vi "Waveform Data Logger Main Page.vi"(8 "error in (no error)":errorcluster, 11 "Node Ptr":T1 format="%.0x") -> (0 "error out":errorcluster)   [LabVIEW 2015, in "Waveform Data Logger System Explorer.lvlib"]
uses:
  Waveform Data Logger System Explorer.lvlib
  <vilib>/NI Veristand/Custom Device API/Custom Device Item Ref.ctl
  Shared/Globals/Global GUIDs.vi
  Shared/Globals/Property Strings.vi
  <vilib>/NI Veristand/Custom Device API/Get Item Property (Boolean).vi
  <vilib>/NI Veristand/Custom Device API/Get Item Property (I32).vi
  <vilib>/NI Veristand/Custom Device Tools/Custom Device Utility Library/NI VeriStand - Search for All Items by GUID.vi
  Shared/Globals/Default Values.vi
  <vilib>/NI Veristand/Custom Device API/Set Item Property (Boolean).vi
  <vilib>/NI Veristand/Custom Device API/Set Item Property (I32).vi
  <vilib>/NI VeriStand/Custom Device API/Custom Device API.lvlib
  <vilib>/NI VeriStand/Custom Device Tools/Custom Device Utility Library/Custom Device Utility Library.lvlib
  Shared/Waveform Data Logger Shared.lvlib
panel:
  in  "Q Size":i32=5 format="%d elements per waveform"
  in  "Auto Q Size":bool
  out "Version":string
  in  "Header 2":cluster{"Section Name":string}={"Section Name"="Waveform Log Files"}
  in  "Remove":bool
  in  "TDMS Log Files":i32(listbox)
  in  "Add File":bool
  in  "Header":cluster{"Section Name":string}={"Section Name"="Waveform Data Logger Specification"}
  out "Name":string
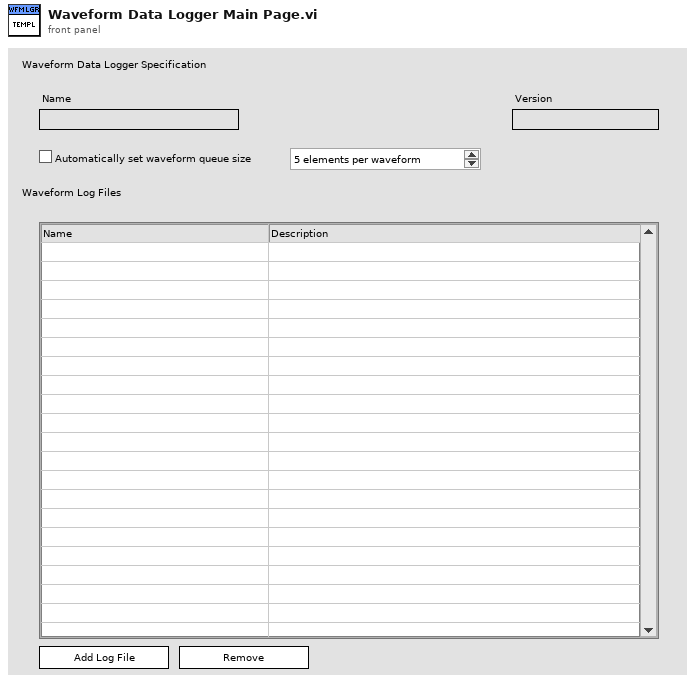
[diagram p1: front panel]
types:
  T1 = typedef "Custom Device API.lvlib/Custom Device Item Ref.ctl" = u64
  T2 = enum8{"Enabled", "Disabled", "Disabled and Grayed Out"}
  T3 = typedef "Custom Device API.lvlib/Custom Device Item Info.ctl" = cluster{"Name":string, "Is Channel":bool, "GUID":string, "Is Waveform":bool}
  T4 = typedef "Custom Device API.lvlib/Custom Device Commands.ctl" = enum16{"Default", "Item renamed", "Shutdown", "Dynamic button pressed"}
  T5 = typedef "LVRowAndColumnTypeDef.ctl" = cluster{"Row":i32, "Column":i32}
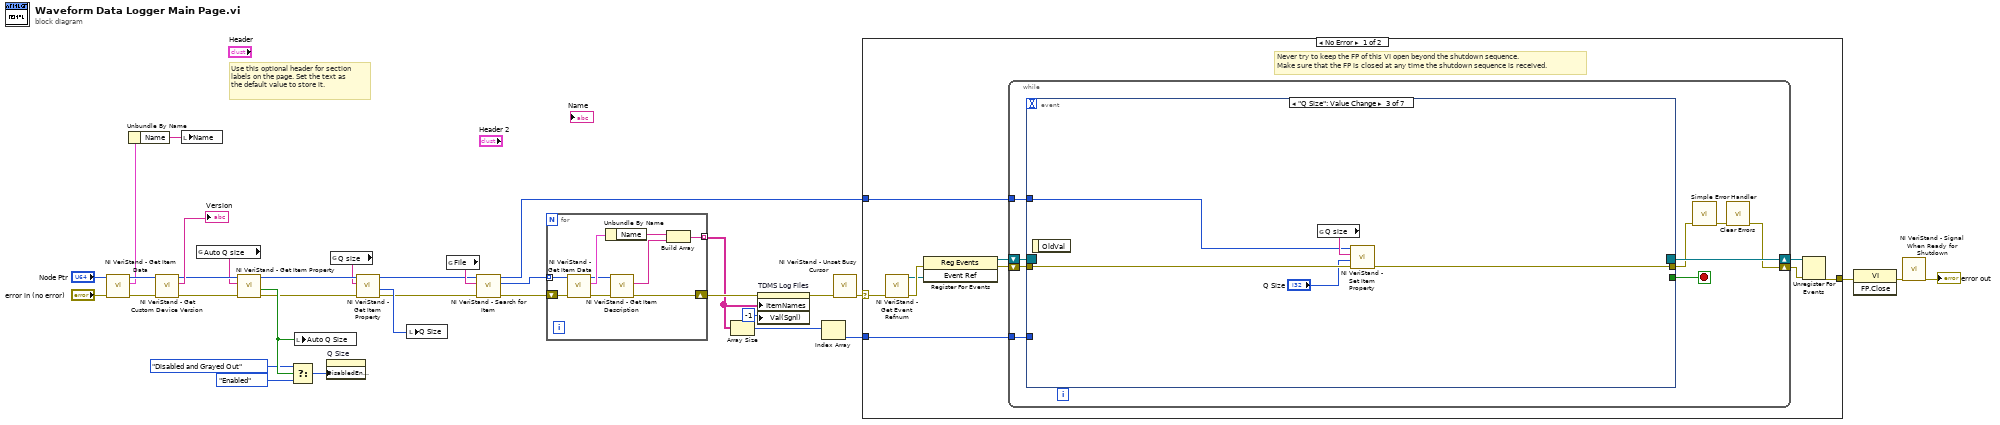
[diagram p0: block diagram]
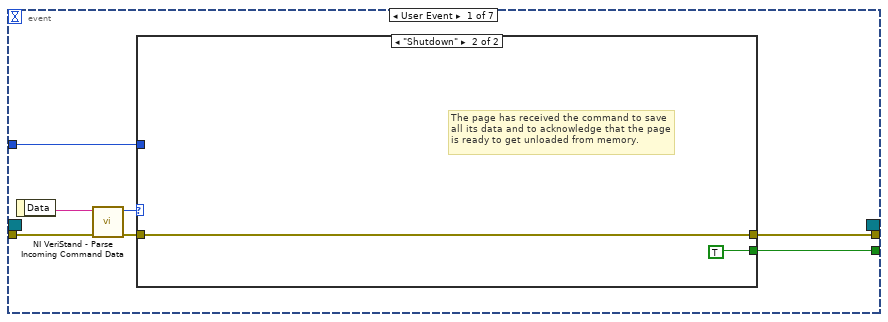
[diagram p2: hidden frame]
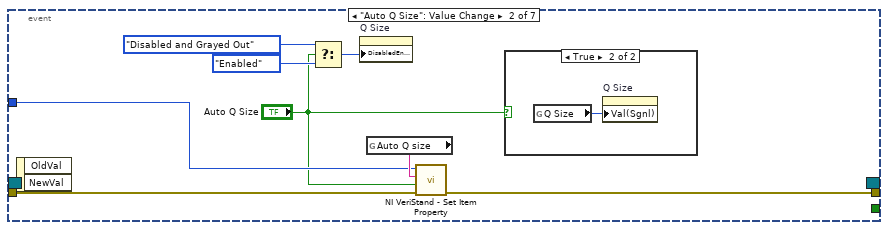
[diagram p4: hidden frame]
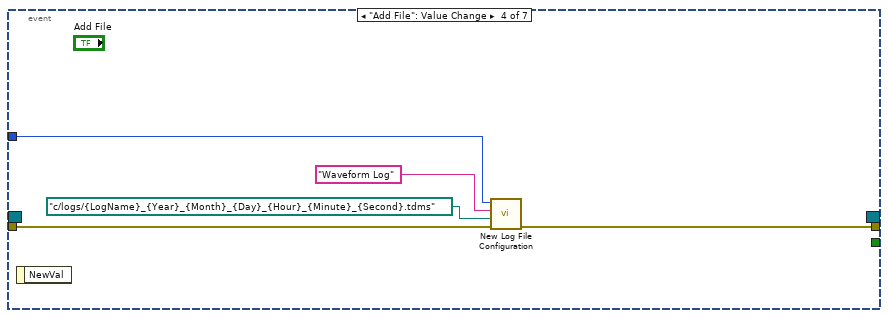
[diagram p6: hidden frame]
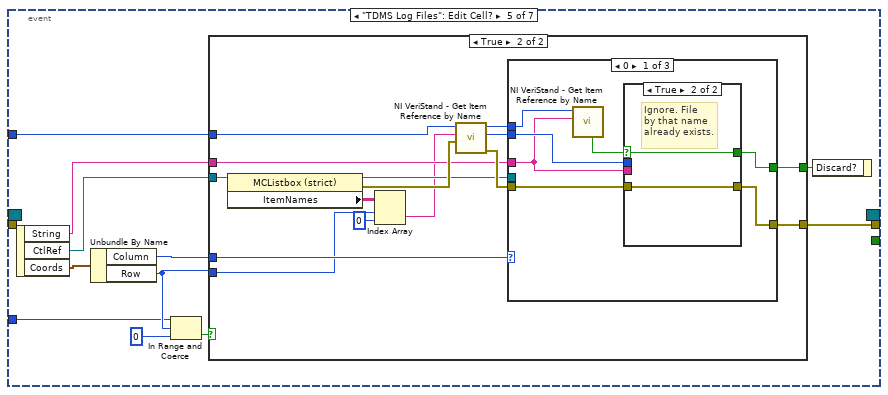
[diagram p7: hidden frame]
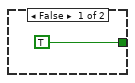
[diagram p8: hidden frame]
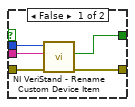
[diagram p9: hidden frame]
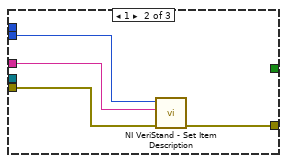
[diagram p10: hidden frame]
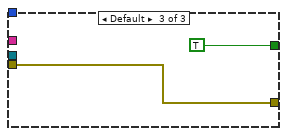
[diagram p11: hidden frame]
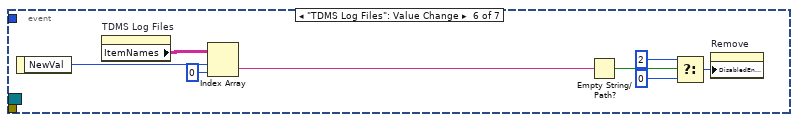
[diagram p12: hidden frame]
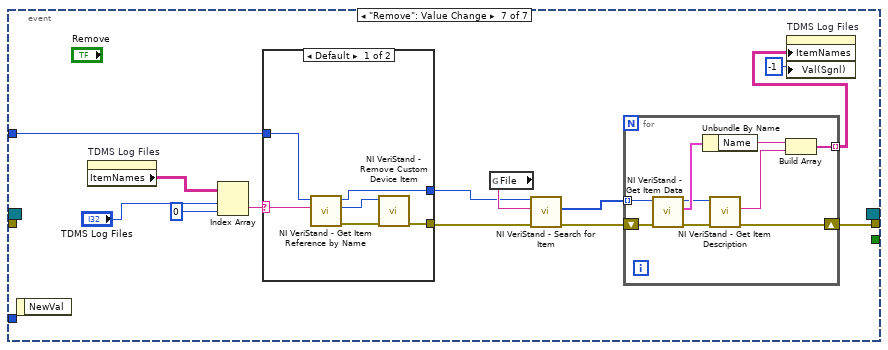
[diagram p13: hidden frame]
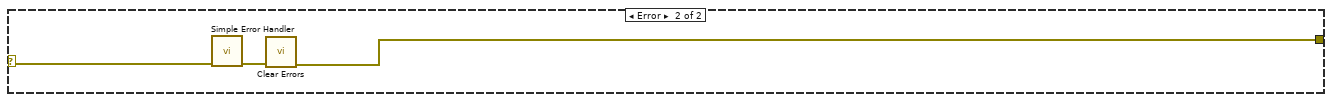
[diagram p15: hidden frame]
diagram:
  # "Use this optional header for section labels on the page. Set the text as the default value to store it."
  n1 = call <vilib>:"NI VeriStand - Get Item Data.vi"("error in (no error)"="error in (no error)", "Item Ref in"="Node Ptr") -> ("error out"=w16:errorcluster, "Item Info"=w1:T3, "Item Ref out"=w17:T1)  [unwired: 7 out]
  n2 = Unbundle By Name(w1) -> ("Name"=w31:string)
  n3 = call <vilib>:"NI VeriStand - Get Custom Device Version.vi"("error in (no error)"=w16, "Device Ref in"=w17) -> ("error out"=w13:errorcluster, "Value"=→"Version":string, "Device Ref out"=w14:T1)  [unwired: 7 in]
  n4 = local write "Name"(w31) -> ()
  n5 = global read "Property Strings.vi" "Auto Q size"() -> (w12:string)
  n6 = call-poly <vilib>:"NI VeriStand - Get Item Property.vi"("error in (no error)"=w13, "Property Name"=w12, "Item Ref in"=w14) -> ("error out"=w6:errorcluster, "Value"=w11:bool, "Item Ref out"=w7:T1)  [unwired: 5 in, 1 out]
  n7 = Select(t=T2."Disabled and Grayed Out" ("Disabled"), s=w11, f=T2."Enabled" ("Disabled")) -> (s? t:f=w8:T2)
  n8 = local write "Auto Q Size"(w11) -> ()
  n9 = property on="Q Size" class="DigNum (strict)"("DisabledEnum"=w8) -> ()  [unwired: 2 in, 2 out]
  n10 = global read "Property Strings.vi" "Q size"() -> (w5:string)
  n11 = call-poly <vilib>:"NI VeriStand - Get Item Property.vi"("error in (no error)"=w6, "Property Name"=w5, "Item Ref in"=w7) -> ("error out"=w3:errorcluster, "Value"=w4:i32, "Item Ref out"=w2:T1)  [unwired: 5 in, 1 out]
  n12 = local write "Q Size"(w4) -> ()
  n13 = global read "Global GUIDs.vi" "File"() -> (w20:string)
  n14 = call-poly <vilib>:"NI VeriStand - Search for Item.vi"("error in"=w3, "Item GUID"=w20, "Section Ref in"=w2) -> ("error out"=w24:errorcluster, "Item Refs"=w23:T1[], "Section Ref out"=w22:T1)  [unwired: 5 in, 1 out]
  n15 = for {
    tunnel: w23 -> [w42] mode=indexing
    tunnel: [w38] -> w27 mode=indexing
    shift-right: [w37] -> w30
    shift-left: w24 -> [w43]
    n16 = call <vilib>:"NI VeriStand - Get Item Data.vi"("error in (no error)"=w43, "Item Ref in"=w42) -> ("error out"=w35:errorcluster, "Item Info"=w41:T3, "Item Ref out"=w36:T1)  [unwired: 6 in, 1 out]
    n17 = Unbundle By Name(w41) -> ("Name"=w40:string)
    n18 = call <vilib>:"NI VeriStand - Get Item Description.vi"("error in (no error)"=w35, "Item Ref in"=w36) -> ("error out"=w37:errorcluster, "Description"=w39:string)  [unwired: 6 in, 2 out]
    n19 = Build Array(w40, w39) -> (w38:string[])
  }
  n20 = Array Size(array=w27) -> (size(s)=w26:i32[])
  n21 = property on="TDMS Log Files" class="MCListbox (strict)"(error in=w30, "ItemNames"=w27, "Val(Sgnl)"=-1 ("Value (Signaling)")) -> (error out=w28:errorcluster)  [unwired: 1 in, 1 out]
  n22 = Index Array(array=w26) -> (element=w25:i32)  [unwired: 1 in]
  n23 = call <vilib>:"NI VeriStand - Unset Busy Cursor.vi"("error in (no error)"=w28) -> ("error out"=w32:errorcluster)  [unwired: 10 out]
  n24 = case shown="No Error" w32 {
    selector: w32 -> [w45 w178]
    tunnel: [w50 w176] -> w19
    tunnel: w22 -> [w46 _]
    tunnel: w25 -> [w44 _]
    frame No Error {
      # "Never try to keep the FP of this VI open beyond the shutdown sequence.\nMake sure that the FP is closed at any time the shutdown sequence is received."
      n25 = call <vilib>:"NI VeriStand - Get Event Refnum.vi"("error in (no error)"=w45) -> ("error out"=w53:errorcluster, "Event Ref"=w49:refnum<user-event>)  [unwired: 9 out]
      n26 = register-events(error in=w53, w49) -> (reference out=w47:refnum<event-registration>, error out=w48:errorcluster)  [unwired: 1 in]
      n27 = while {
        tunnel: w46 -> [w59]
        shift-right: [w56] -> w51
        shift-left: w48 -> [w61]
        shift-right: [w62] -> w52
        shift-left: w47 -> [w54]
        tunnel: w44 -> [w55]
        stop <- w60 stop-if-true
        n28 = event shown="[2] \"Q Size\": Value Change" {
          selector: w54 -> [_ _ _ _ _ _ _]
          dyn-events: [_ _ _ _ _ _ _] -> w62
          timeout: _ -> [_ _ _ _ _ _ _]
          tunnel: w61 -> [w69 w79 w84 w90 _ _ _]
          tunnel: [w65 _ _ _ _ _ _] -> w60
          tunnel: [w64 w77 w82 w89 w98 _ w149] -> w58
          tunnel: w59 -> [w63 w78 w85 w91 w93 _ w157]
          tunnel: w55 -> [_ _ _ _ w92 _ _]
          event User Event {
            n29 = event-data() -> ("Data"=w68:string)  [unwired: 1 out]
            n30 = call <vilib>:"NI VeriStand - Parse Incoming Command Data.vi"("error in (no error)"=w69, "Incoming data"=w68) -> ("error out"=w67:errorcluster, "Action"=w66:T4)  [unwired: 8 out]
            n31 = case shown="\"Shutdown\"" w66 {
              tunnel: w67 -> [w70 w71]
              tunnel: [_ TRUE] -> w65
              tunnel: [w70 w71] -> w64
              tunnel: w63 -> [_ _]
              frame "Default", Default {
              }
              frame "Shutdown" {
                # "The page has received the command to save all its data and to acknowledge that the page is ready to get unloaded from memory."
              }
            }
          }
          event "Auto Q Size": Value Change {
            n32 = event-data() -> ()  [unwired: 3 out]
            n33 = Select(t=T2."Disabled and Grayed Out" ("Disabled"), s="Auto Q Size", f=T2."Enabled" ("Disabled")) -> (s? t:f=w76:T2)
            n34 = property on="Q Size" class="DigNum (strict)"("DisabledEnum"=w76) -> ()  [unwired: 2 in, 2 out]
            n35 = global read "Property Strings.vi" "Auto Q size"() -> (w80:string)
            n36 = call-poly <vilib>:"NI VeriStand - Set Item Property.vi"("error in (no error)"=w79, "Value"="Auto Q Size", "Property Name"=w80, "Item Ref in"=w78) -> ("error out"=w77:errorcluster)  [unwired: 5 in, 2 out]
            n37 = case shown="True" "Auto Q Size" {
              frame False {
              }
              frame True {
                n38 = global read "Default Values.vi" "Q Size"() -> (w81:i32)
                n39 = property on="Q Size" class="DigNum (strict)"("Val(Sgnl)"=w81) -> ()  [unwired: 2 in, 2 out]
              }
            }
          }
          event "Q Size": Value Change {
            n40 = event-data() -> ()  [unwired: 2 out]
            n41 = global read "Property Strings.vi" "Q size"() -> (w86:string)
            n42 = call-poly <vilib>:"NI VeriStand - Set Item Property.vi"("error in (no error)"=w84, "Value"="Q Size", "Property Name"=w86, "Item Ref in"=w85) -> ("error out"=w82:errorcluster)  [unwired: 5 in, 2 out]
          }
          event "Add File": Value Change {
            n43 = event-data() -> ()  [unwired: 2 out]
            n44 = call "New Log File Configuration.vi"("error in (no error)"=w90, "Default Path"=path "c:/logs/{LogName}_{Year}_{Month}_{Day}_{Hour}_{Minute}_{Second}.tdms" ("Default Log Directory"), "Default Name"="Waveform Log", "Device Ref in"=w91) -> ("error out"=w89:errorcluster)  [unwired: 7 out]
          }
          event "TDMS Log Files": Edit Cell? {
            n45 = event-data() -> ("String"=w95:string, "CtlRef"=w94:refnum<vi>, "Coords"=w96:T5)  [unwired: 1 out]
            n46 = Unbundle By Name(w96) -> ("Column"=w102:i32, "Row"=w100:i32)
            n47 = In Range and Coerce(upper limit=w92, x=w100, lower limit=0) -> (In Range?=w99:bool)  [unwired: 1 out]
            n48 = case shown="True" w99 {
              tunnel: w94 -> [_ w116]
              tunnel: [TRUE w113] -> w97
              tunnel: w95 -> [_ w111]
              tunnel: w93 -> [_ w109]
              tunnel: w100 -> [_ w108]
              tunnel: w102 -> [_ w114]
              tunnel: [_ w110] -> w98
              frame False {
              }
              frame True {
                n49 = property class="MCListbox (strict)"(reference=w116) -> (reference out=w112:refnum<vi>, error out=w118:errorcluster, "ItemNames"=w115:string[][])  [unwired: 1 in]
                n50 = Index Array(array=w115, index (row)=w108, index (col)=0 ("disabled index (col)")) -> (element=w106:string)
                n51 = call <vilib>:"NI VeriStand - Get Item Reference by Name.vi"("error in (no error)"=w118, "Item Name"=w106, "Parent Ref in"=w109) -> ("error out"=w117:errorcluster, "Item Ref"=w105:T1, "Parent Ref out"=w104:T1)  [unwired: 5 in, 1 out]
                n52 = case shown="0" w114 {
                  tunnel: [w119 _ TRUE] -> w113
                  tunnel: w105 -> [w124 w135 _]
                  tunnel: w117 -> [w125 w133 w137]
                  tunnel: w112 -> [_ _ _]
                  tunnel: w111 -> [w121 w134 _]
                  tunnel: [w123 w136 w137] -> w110
                  tunnel: w104 -> [w122 _ _]
                  frame 0 {
                    n53 = call <vilib>:"NI VeriStand - Get Item Reference by Name.vi"("Item Name"=w121, "Parent Ref in"=w122) -> ("Found"=w120:bool)  [unwired: 6 in, 3 out]
                    n54 = case shown="True" w120 {
                      selector: w120 -> [_ w131]
                      tunnel: w125 -> [w130 w132]
                      tunnel: w124 -> [w129 _]
                      tunnel: [w128 w132] -> w123
                      tunnel: w121 -> [w127 _]
                      tunnel: [w126 w131] -> w119
                      frame False {
                        n55 = call <vilib>:"NI VeriStand - Rename Custom Device Item.vi"("error in (no error)"=w130, "New Name"=w127, "Item Ref in"=w129) -> ("error out"=w128:errorcluster, "Request invalid?"=w126:bool)  [unwired: 6 in, 1 out]
                      }
                      frame True {
                        # "Ignore. File\nby that name\nalready exists."
                      }
                    }
                  }
                  frame 1 {
                    n56 = call <vilib>:"NI VeriStand - Set Item Description.vi"("error in (no error)"=w133, "Description"=w134, "Item Ref in"=w135) -> ("error out"=w136:errorcluster)  [unwired: 6 in, 2 out]
                  }
                  frame Default {
                  }
                }
              }
            }
            n57 = event-data("Discard?"=w97) -> ()  [unwired: 1 in, 1 out]
          }
          event "TDMS Log Files": Value Change {
            n58 = event-data() -> ("NewVal"=w139:i32)  [unwired: 1 out]
            n59 = property on="TDMS Log Files" class="MCListbox (strict)"() -> ("ItemNames"=w140:string[][])  [unwired: 2 in, 2 out]
            n60 = Index Array(array=w140, index (row)=w139, index (col)=0 ("disabled index (col)")) -> (element=w143:string)
            n61 = Empty String/Path?(string/path=w143) -> (empty?=w142:bool)
            n62 = Select(t=u8 2, s=w142, f=u8 0) -> (s? t:f=w144:u8)
            n63 = property on="Remove" class="Bool"("DisabledEnum"=w144) -> ()  [unwired: 2 in, 2 out]
          }
          event "Remove": Value Change {
            n64 = event-data() -> ()  [unwired: 2 out]
            n65 = property on="TDMS Log Files" class="MCListbox (strict)"() -> ("ItemNames"=w156:string[][])  [unwired: 2 in, 2 out]
            n66 = Index Array(array=w156, index (row)="TDMS Log Files", index (col)=0 ("disabled index (col)")) -> (element=w159:string)
            n67 = case shown="Default" w159 {
              selector: w159 -> [w171 _]
              tunnel: w157 -> [w172 w175]
              tunnel: [w174 _] -> w148
              tunnel: [w169 w175] -> w147
              frame Default {
                n68 = call <vilib>:"NI VeriStand - Get Item Reference by Name.vi"("Item Name"=w171, "Parent Ref in"=w172) -> ("error out"=w173:errorcluster, "Item Ref"=w170:T1, "Parent Ref out"=w169:T1)  [unwired: 6 in, 1 out]
                n69 = call <vilib>:"NI VeriStand - Remove Custom Device Item.vi"("error in (no error)"=w173, "Item Ref in"=w170) -> ("error out"=w174:errorcluster)  [unwired: 8 in, 1 out]
              }
              frame "" {
              }
            }
            n70 = global read "Global GUIDs.vi" "File"() -> (w152:string)
            n71 = call-poly <vilib>:"NI VeriStand - Search for Item.vi"("error in"=w148, "Item GUID"=w152, "Section Ref in"=w147) -> ("error out"=w154:errorcluster, "Item Refs"=w153:T1[])  [unwired: 5 in, 2 out]
            n72 = for {
              tunnel: w153 -> [w167] mode=indexing
              tunnel: [w163] -> w150 mode=indexing
              shift-right: [w162] -> w149
              shift-left: w154 -> [w168]
              n73 = call <vilib>:"NI VeriStand - Get Item Data.vi"("error in (no error)"=w168, "Item Ref in"=w167) -> ("error out"=w160:errorcluster, "Item Info"=w166:T3, "Item Ref out"=w161:T1)  [unwired: 6 in, 1 out]
              n74 = Unbundle By Name(w166) -> ("Name"=w165:string)
              n75 = call <vilib>:"NI VeriStand - Get Item Description.vi"("error in (no error)"=w160, "Item Ref in"=w161) -> ("error out"=w162:errorcluster, "Description"=w164:string)  [unwired: 6 in, 2 out]
              n76 = Build Array(w165, w164) -> (w163:string[])
            }
            n77 = property on="TDMS Log Files" class="MCListbox (strict)"("ItemNames"=w150, "Val(Sgnl)"=-1 ("Value (Signaling)")) -> ()  [unwired: 2 in, 2 out]
          }
        }
        n78 = call <vilib>:"Simple Error Handler.vi"("error in (no error)"=w58) -> ("error out"=w57:errorcluster)  [unwired: 1 in, 7 out]
        n79 = call <vilib>:"Clear Errors.vi"("error in (no error)"=w57) -> ("error out"=w56:errorcluster)  [unwired: 1 in, 5 out]
      }
      n80 = Unregister For Events(event registration refnum=w52, error in=w51) -> (error out=w50:errorcluster)
    }
    frame Error {
      n81 = call <vilib>:"Simple Error Handler.vi"("error in (no error)"=w178) -> ("error out"=w177:errorcluster)  [unwired: 1 in, 7 out]
      n82 = call <vilib>:"Clear Errors.vi"("error in (no error)"=w177) -> ("error out"=w176:errorcluster)  [unwired: 1 in, 5 out]
    }
  }
  n83 = invoke class="VI" method="FP.Close"(error in=w19) -> (error out=w34:errorcluster)  [unwired: 2 in, 2 out]
  n84 = call <vilib>:"NI VeriStand - Signal When Ready for Shutdown.vi"("error in (no error)"=w34) -> ("error out"=→"error out":errorcluster)  [unwired: 10 out]
